vi "Configure Settings.vi"(8 "Error In":errorcluster, 11 "Refnums":T5) -> (0 "Error Out":errorcluster, 1 "Cancelled?":bool, 2 "Recording Settings Out":T1={"Folder to Save Recordings"=path "", "Video FPS"=5, "Codec"=3, "Tracker FPS"=40, "Operator ID"={"Operator ID"=0, "Expertise"=0}, "Patient ID/Gestation"={"ID"=0, "Gestation"=""}} {"Patient ID/Gestation"."ID" format="%0#3.2f"; "Operator ID"."Operator ID" format="%03.0f"; "Operator ID"."Expertise" items=["Novice", "Expert"]; "Tracker FPS" max=100; "Codec" items=["Cinepak Codec by Radius", "Intel IYUV codec", "Microsoft Video 1", "FF Video Codec 1 (FFV1) (NI Vision)", "Motion JPEG (NI Vision)", "Y800 Uncompressed Grey Scale (NI Vision)", "YUV 4:2:0 Planar (NI Vision)"]; "Video FPS" max=100}, 3 "Connection Settings Out":T6={"Frame Grabber"="cam1", "Tracker"=enum."Aurora", "Port"=enum."COM1"} caption="These settings must be set BEFORE running the program!")   [LabVIEW 2017]
uses:
  Controls/Connection Settings.ctl
  <vilib>/userdefined/High Color/IMAQdx.ctl
  Controls/Tracker Type.ctl
  Controls/COM Port.ctl
  Controls/Refnums.ctl
  Controls/Recording Settings.ctl
  Controls/Operator Settings.ctl
  Controls/Operator.ctl
  Controls/Patient Settings.ctl
panel:
  in  "Recording Settings":T1={"Folder to Save Recordings"=path "", "Video FPS"=5, "Codec"=3, "Tracker FPS"=40, "Operator ID"={"Operator ID"=0, "Expertise"=0}, "Patient ID/Gestation"={"ID"=0, "Gestation"=""}} {"Patient ID/Gestation"."ID" format="%0#3.2f"; "Operator ID"."Operator ID" format="%03.0f"; "Operator ID"."Expertise" items=["Novice", "Expert"]; "Tracker FPS" max=100; "Codec" items=["Cinepak Codec by Radius", "Intel IYUV codec", "Microsoft Video 1", "FF Video Codec 1 (FFV1) (NI Vision)", "Motion JPEG (NI Vision)", "Y800 Uncompressed Grey Scale (NI Vision)", "YUV 4:2:0 Planar (NI Vision)"]; "Video FPS" max=100}
  in  "Cancel":bool
  in  "Connection Settings":T6={"Frame Grabber"="cam1", "Tracker"=enum."Aurora", "Port"=enum."COM1"} caption="These settings must be set BEFORE running the program!"
  in  "OK":bool
  # "US Probe should always \nbe 1st tool\n\nOptiTrack assumes two tracked objects and computes  position of probe relative\nto phantom"
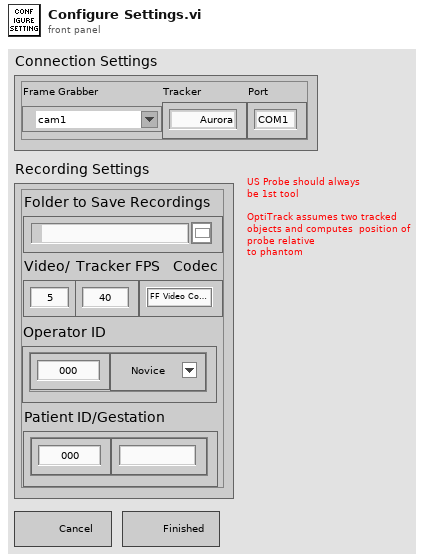
[diagram p1: front panel]
types:
  T1 = typedef "Recording Settings.ctl" = cluster{"Folder to Save Recordings":path, "Video FPS":u32, "Codec":u16, "Tracker FPS":u32, "Operator ID":T2, "Patient ID/Gestation":T4}
  T2 = typedef "Operator Settings.ctl" = cluster{"Operator ID":u32, "Expertise":T3}
  T3 = typedef "Operator.ctl" = u16
  T4 = typedef "Patient Settings.ctl" = cluster{"ID":u32, "Gestation":string}
  T5 = typedef "Refnums.ctl" = cluster{"Live Refnum":refnum<vi>, "Record Refnum":refnum<vi>, "Playback Refnum":refnum<vi>, "Frame Slider Refnum":refnum<vi>, "Pause Refnum":refnum<vi>, "Home Refnum":refnum<vi>, "Set Crop Refnum":refnum<vi>, "Clear Crop Refnum":refnum<vi>, "stop refnum":refnum<vi>, "Playback Rate Refnum":refnum<vi>, "Presentation Refnum":refnum<vi>, "Crop Time Frame Slider Refnum":refnum<vi>, "Cancel Save Refnum":refnum<vi>, "Reverse Playback Refnum":refnum<vi>, "Recording Settings Refnum":refnum<vi>, "Continuous Playback Refnum":refnum<vi>, "Annotation Refnum":refnum<vi>, "Export All Refnum":refnum<vi>, "Export List Refnum":refnum<vi>, "Fill List Refnum":refnum<vi>, "Save Crop Refnum":refnum<vi>, "Skip Forward Refnum":refnum<vi>, "Skip Backward Refnum":refnum<vi>, "Single Annotation Refnum":refnum<vi>, "Load Video Refnum":refnum<vi>, "Set Start Refnum":refnum<vi>, "Set End Refnum":refnum<vi>, "Add to List Refnum":refnum<vi>, "List of Annotations Refnum":refnum<vi>, "Camera Frame Refnum":refnum<vi>, "Load Image Refnum":refnum<vi>, "Saving Refnum":refnum<vi>}
  T6 = typedef "Connection Settings.ctl" = cluster{"Frame Grabber":T7, "Tracker":T8, "Port":T9}
  T7 = typedef "IMAQdx.ctl" = refnum<k21>
  T8 = typedef "Tracker Type.ctl" = enum16{"Aurora", "OptiTrack"}
  T9 = typedef "COM Port.ctl" = enum16{"COM1", "COM2", "COM3", "COM4", "COM5", "COM6", "COM7", "COM8", "COM9", "COM10", "COM11", "COM12", "COM13", "COM14", "COM15", "COM16", "COM17", "COM18", "COM19", "COM20"}
  T10 = enum8{"Enabled", "Disabled", "Disabled and Grayed Out"}
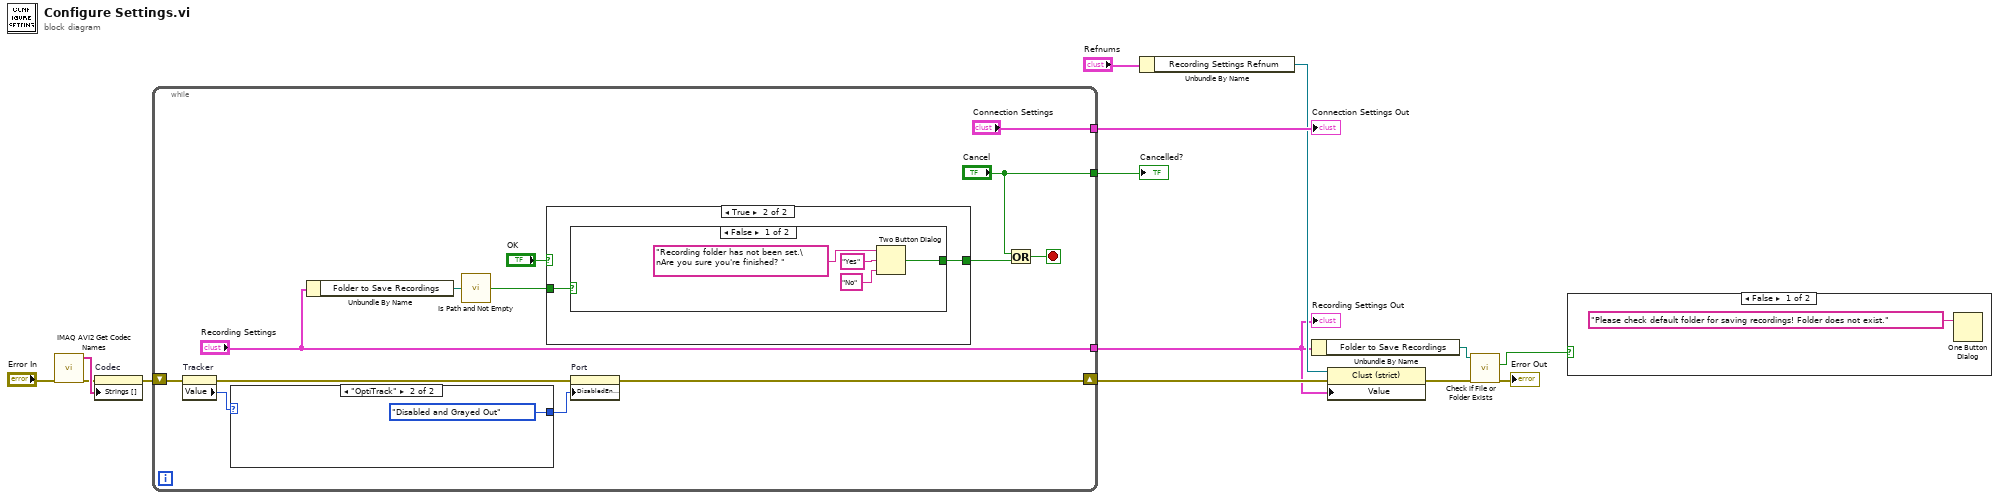
[diagram p0: block diagram]
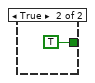
[diagram p4: hidden frame]
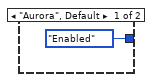
[diagram p5: hidden frame]
diagram:
  n1 = call "IMAQ AVI2 Get Codec Names"("error in (no error)"="Error In") -> ("error out"=w2:errorcluster, "Codec Names"=w3:string[])  [unwired: 9 in]
  n2 = property on="Codec" class="Ring (strict)"(error in=w2, "Strings []"=w3) -> (error out=w1:errorcluster)  [unwired: 1 in, 1 out]
  n3 = while {
    shift-right: [w15] -> w12
    shift-left: w1 -> [w24]
    tunnel: ["Connection Settings"] -> w14
    tunnel: ["Recording Settings"] -> w5
    tunnel: ["Cancel"] -> w11
    stop <- w26 stop-if-true
    n4 = property on="Tracker" class="Enum (strict)"(error in=w24) -> (error out=w23:errorcluster, "Value"=w22:T8)  [unwired: 1 in, 1 out]
    n5 = case shown="\"OptiTrack\"" w22 {
      tunnel: [T10."Enabled" ("Disabled") T10."Disabled and Grayed Out" ("Disabled")] -> w21
      frame "Aurora", Default {
      }
      frame "OptiTrack" {
      }
    }
    n6 = Unbundle By Name("Recording Settings") -> ("Folder to Save Recordings"=w19:path)
    n7 = call <vilib>:"Is Path and Not Empty.vi"("path"=w19) -> ("Is Path and Not Empty?"=w16:bool)  [unwired: 4 in]
    n8 = case shown="True" "OK" {
      selector: "OK" -> [w28 _]
      tunnel: [w28 w29] -> w18
      tunnel: w16 -> [_ w30]
      frame False {
      }
      frame True {
        n9 = case shown="False" w30 {
          tunnel: [w31 TRUE ("T button?")] -> w29
          frame False {
            n10 = Two Button Dialog(message="Recording folder has not been set.\nAre you sure you're finished? ", 1:"No" ("F button name (\"Cancel\")"), 2:"Yes" ("T button name (\"OK\")")) -> (T button?=w31:bool)
          }
          frame True {
          }
        }
      }
    }
    n11 = property on="Port" class="Enum (strict)"(error in=w23, "DisabledEnum"=w21) -> (error out=w15:errorcluster)  [unwired: 1 in, 1 out]
    n12 = Or(x="Cancel", y=w18) -> (x .or. y?=w26:bool)
  }
  "Connection Settings Out" <- w14
  "Recording Settings Out" <- w5
  "Cancelled?" <- w11
  n13 = Unbundle By Name("Refnums") -> ("Recording Settings Refnum"=w6:refnum<vi>)
  n14 = Unbundle By Name(w5) -> ("Folder to Save Recordings"=w10:path)
  n15 = property class="Clust (strict)"(reference=w6, error in=w12, "Value"=w5) -> (error out=w8:errorcluster)  [unwired: 1 out]
  n16 = call <vilib>:"Check if File or Folder Exists.vi"("error in (no error)"=w8, "path"=w10) -> ("error out"=→"Error Out":errorcluster, "file or folder exists?"=w9:bool)  [unwired: 7 in, 1 out]
  n17 = case shown="False" w9 {
    frame False {
      n18 = One Button Dialog(message="Please check default folder for saving recordings! Folder does not exist.") -> ()  [unwired: 1 in, 1 out]
    }
    frame True {
    }
  }
